vi "PicoScope6000aClose.vi"(8 "error in (no error)":errorcluster, 11 "handle in":i16=16384) -> (0 "error out":errorcluster, 3 "handle out":i16)   [LabVIEW 2010]
doc: "This closes the device and should be called before exiting an application."
uses:
  ps6000a.dll
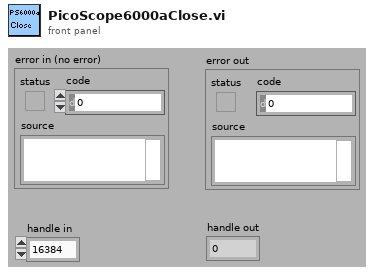
[diagram p1: front panel]
types:
  T1 = cluster{"status":bool, "code":u32, "source":string}
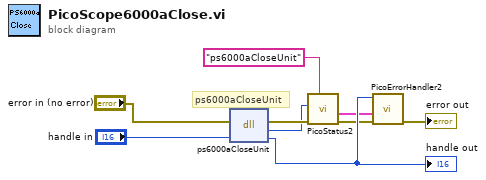
[diagram p0: block diagram]
diagram:
  # "ps6000aCloseUnit"
  n1 = dll-call lib="ps6000a.dll" fn="ps6000aCloseUnit"(error in="error in (no error)", "handle"="handle in") -> (error out=w2:errorcluster, "PICO_STATUS"=w1:u32, "handle"=w6:i16)  [unwired: 2 in, 1 out]
  "handle out" <- w6
  n2 = call "PicoStatus2.vi"("PICO source"="ps6000aCloseUnit" ("source"), "Error in"=w2, "PICO STATUS"=w1) -> ("error out"=w5:errorcluster, "PICO_STATUS out"=w4:T1)  [unwired: 5 in]
  n3 = call "PicoErrorHandler2.vi"("error in (no error)"=w5, "PICO_STATUS in"=w4, "handle In"=w6) -> ("error out"=→"error out":errorcluster)  [unwired: 8 in]
